vi "PCO_Live.vi"(7 "Message Data":variant, 8 "entrée d'erreur (pas d'erreur)":errorcluster, 9 "Display loop":refnum<queue>, 10 "dup Message Queue":refnum<queue>, 11 "Camera en entrée":refnum<class "Camera.lvclass">) -> (0 "sortie d'erreur":errorcluster, 3 "Camera en sortie":refnum<class "Camera.lvclass">)   [LabVIEW 2026]
uses:
  v0.2/SubVIs/QMH/Message Queue/Message Cluster.ctl
  <instrlib>/PCO_SDK/File Group 0/vi.lib/Excelitas PCO GmbH/pco.labview/camera/Camera.lvclass
  v0.2/SubVIs/Controls/PCO_Config.ctl
  v0.2/SubVIs/Controls/TypeDef_FGV.ctl
  <instrlib>/PCO_SDK/File Group 0/vi.lib/Excelitas PCO GmbH/pco.labview/camera/Controls/binning.ctl
  v0.2/SubVIs/QMH/Message Queue/Enqueue Message (Single).vi
  v0.2/SubVIs/QMH/Message Queue/Message Queue.lvlib
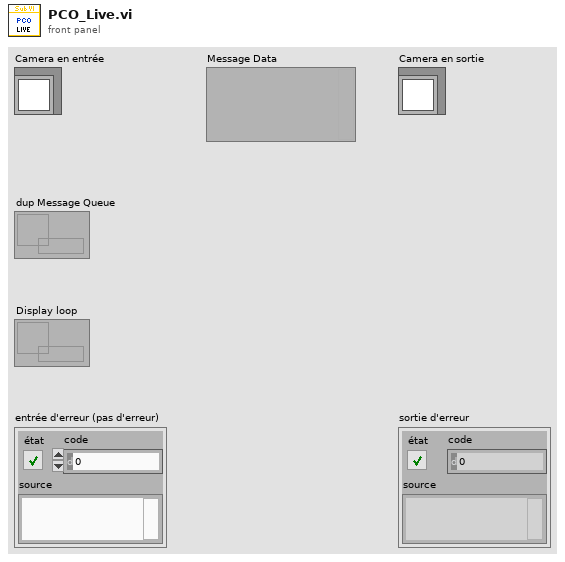
[diagram p1: front panel]
types:
  T1 = typedef "PCO_Config.ctl" = cluster{"Exposure time (s)":dbl, "TriggerMode":u16, "ROI X0":u16, "ROI Y0":u16, "ROI X1":u16, "ROI Y1":u16, "Binning":u8}
  T2 = enum16{"sequence", "sequence non blocking", "ring buffer", "fifo", "sequence_dpcore", "sequence_non_blocking_dpcore", "ring_buffer_dpcore", "fifo_dpcore", "tif", "multitif", "pcoraw", "b16", "dicom", "multidicom", "camram_ring", "camram_segment"}
  T3 = typedef "Camera.lvclass/binning.ctl" = cluster{"vert":u16, "horz":u16, "mode":u16}
  T4 = cluster{"exposure_time_s":dbl, "delay_time_s":dbl, "roi":cluster{"x0":u64, "y0":u64, "x1":u64, "y1":u64}, "timestamp_mode":u16, "pixelrate":u32, "trigger_mode":u16, "acquire_mode":u16, "metadata_mode":u16, "noisefilter_mode":u16, "pixel_format":u32, "binning":T3, "auto_exposure":cluster{"region":u16, "min_exposure_s":dbl, "max_exposure_s":dbl}}
  T5 = typedef "TypeDef_FGV.ctl" = enum16{"Initialize", "Write", "Read"}
  T6 = enum16{"Undefined", "Mono8", "Mono16", "BGRA8", "RGBA8", "BGRA16", "RGBA16", "CompressedMono8"}
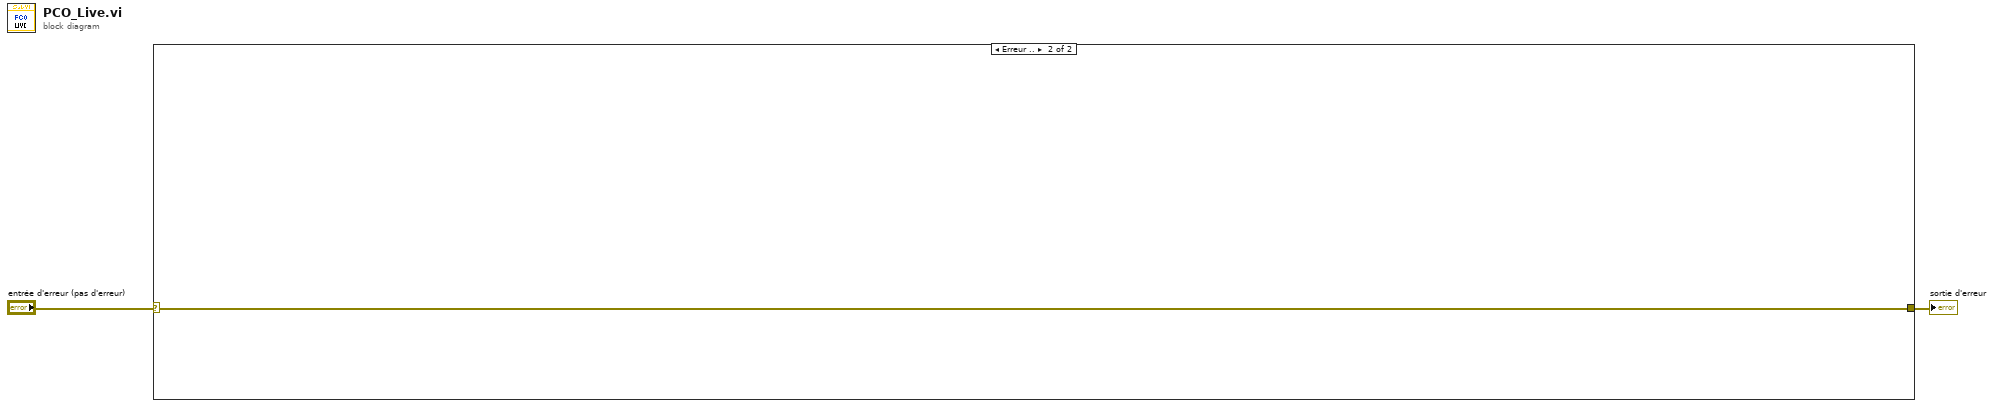
[diagram p0: block diagram]
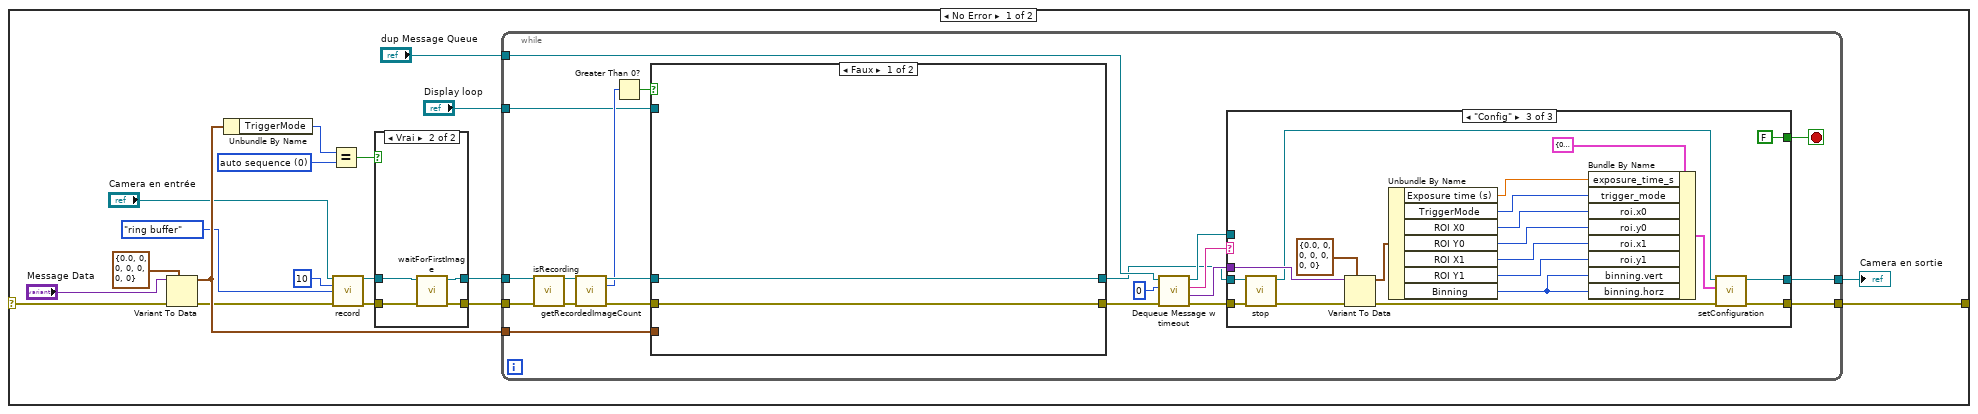
[diagram p2: hidden frame]
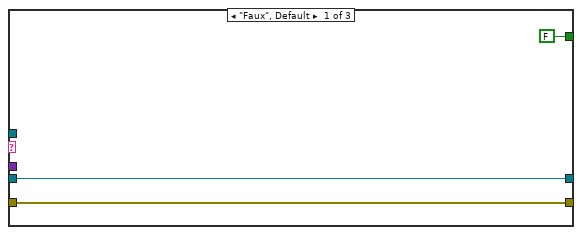
[diagram p3: hidden frame]
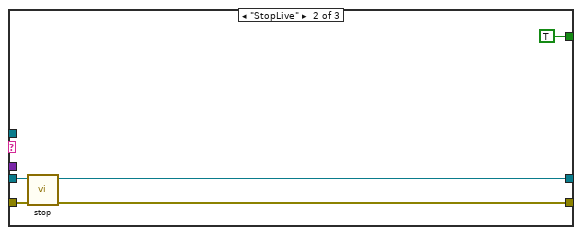
[diagram p4: hidden frame]
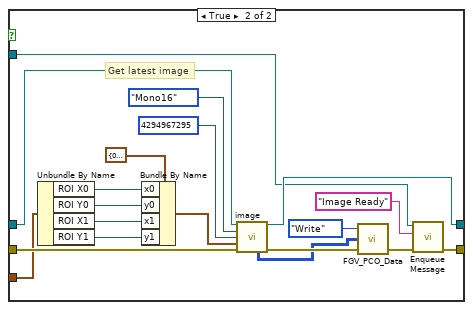
[diagram p5: hidden frame]
diagram:
  n1 = case shown="Erreur .." "entrée d'erreur (pas d'erreur)" {
    selector: "entrée d'erreur (pas d'erreur)" -> [w3 w98]
    tunnel: [w17 w98] -> w2
    frame No Error {
      w9 = u16 0 items=["auto sequence", "software trigger", "external exposure start", "external exposure control"] ("TriggerMode")
      n2 = Variant To Data(error in=w3, type=T1 {"Exposure time (s)"=0.0, "TriggerMode"=0, "ROI X0"=0, "ROI Y0"=0, "ROI X1"=0, "ROI Y1"=0, "Binning"=0} ("PCO_Config"), Variant="Message Data") -> (data=w15:T1, error out=w8:errorcluster)
      n3 = Unbundle By Name(w15) -> ("TriggerMode"=w10:u16)
      n4 = Equal?(x=w10, y=w9) -> (x = y?=w12:bool)
      n5 = call-dynamic "record.vi"("Camera in"="Camera en entrée", "num_images"=u32 10 ("dwImgCount"), "record_mode"=T2."ring buffer", "error in (no error)"=w8) -> ("Camera out"=w20:refnum<class "Camera.lvclass">, "error out"=w19:errorcluster)  [unwired: 10 in]
      n6 = case shown="Vrai" w12 {
        tunnel: w19 -> [w92 w97]
        tunnel: w20 -> [w93 w96]
        tunnel: [w93 w95] -> w14
        tunnel: [w92 w94] -> w13
        frame False {
        }
        frame True {
          n7 = call-dynamic "waitForFirstImage.vi"("error in (no error)"=w97, "Camera in"=w96) -> ("error out"=w94:errorcluster, "Camera out"=w95:refnum<class "Camera.lvclass">)  [unwired: 8 in]
        }
      }
      n8 = while {
        tunnel: w13 -> [w36]
        tunnel: w14 -> [w35]
        tunnel: w15 -> [w34]
        tunnel: "dup Message Queue" -> [w32]
        tunnel: "Display loop" -> [w30]
        tunnel: [w25] -> w17
        tunnel: [w24] -> w18
        stop <- w23 stop-if-true
        n9 = call-dynamic "isRecording.vi"("Camera in"=w35, "error in (no error)"=w36) -> ("Camera out"=w42:refnum<class "Camera.lvclass">, "error out"=w41:errorcluster)  [unwired: 11 in, 1 out]
        n10 = call-dynamic "getRecordedImageCount.vi"("Camera in"=w42, "error in (no error)"=w41) -> ("Camera out"=w39:refnum<class "Camera.lvclass">, "recorded_image_count"=w37:u32, "error out"=w40:errorcluster)  [unwired: 11 in]
        n11 = Greater Than 0?(x=w37) -> (x > 0?=w38:bool)
        n12 = case shown="Faux" w38 {
          tunnel: [w71 w77] -> w33
          tunnel: w40 -> [w71 w88]
          tunnel: w39 -> [w72 w87]
          tunnel: [w72 w86] -> w26
          tunnel: w34 -> [_ w85]
          tunnel: w30 -> [_ w79]
          frame False {
          }
          frame True {
            # "Get latest image"
            n13 = Unbundle By Name(w85) -> ("ROI X0"=w84:u16, "ROI Y0"=w83:u16, "ROI X1"=w82:u16, "ROI Y1"=w81:u16)
            n14 = Bundle By Name(cluster=cluster{"x0":u64, "y0":u64, "x1":u64, "y1":u64} {"x0"=0, "y0"=0, "x1"=0, "y1"=0} ("roi"), "x0"=w84, "y0"=w83, "x1"=w82, "y1"=w81) -> (w89:cluster{"x0":u64, "y0":u64, "x1":u64, "y1":u64})
            n15 = call-dynamic "image.vi"("Camera in"=w87, "data_format"=T6."Mono16", "image_index"=u32 4294967295 ("dwImgIdx"), "roi"=w89, "error in (no error)"=w88) -> ("Camera out"=w86:refnum<class "Camera.lvclass">, "raw_image (U16)"=w73:u16[][], "error out"=w75:errorcluster)  [unwired: 2 in, 6 out]
            n16 = call "FGV_PCO_Data.vi"("error in"=w75, "Data"=w73, "Action"=TypeDef_FGV."Write") -> ("error out"=w74:errorcluster)  [unwired: 1 in, 1 out]
            n17 = call-poly "Enqueue Message.vi"("error in (no error)"=w74, "Message"="Image Ready", "Message Queue"=w79) -> ("error out"=w77:errorcluster)  [unwired: 7 in, 1 out]
          }
        }
        n18 = call "Dequeue Message w timeout.vi"("entrée d'erreur (pas d'erreur)"=w33, "timeout en ms (-1)"=0, "Message Queue"=w32) -> ("sortie d'erreur"=w28:errorcluster, "Message Data"=w27:variant, "Message"=w31:string, "Message Queue"=w29:refnum<queue>)  [unwired: 5 in]
        n19 = case shown="\"Config\"" w31 {
          tunnel: w29 -> [_ _ _]
          tunnel: w28 -> [w44 w49 w69]
          tunnel: w27 -> [_ _ w55]
          tunnel: w26 -> [w45 w50 w70]
          tunnel: [w44 w48 w51] -> w25
          tunnel: [w45 w47 w53] -> w24
          tunnel: [FALSE TRUE FALSE] -> w23
          frame "Faux", Default {
          }
          frame "StopLive" {
            n20 = call-dynamic "stop.vi"("error in (no error)"=w49, "Camera in"=w50) -> ("error out"=w48:errorcluster, "Camera out"=w47:refnum<class "Camera.lvclass">)  [unwired: 8 in]
          }
          frame "Config" {
            n21 = call-dynamic "stop.vi"("error in (no error)"=w69, "Camera in"=w70) -> ("error out"=w54:errorcluster, "Camera out"=w52:refnum<class "Camera.lvclass">)  [unwired: 8 in]
            n22 = Variant To Data(error in=w54, type=T1 {"Exposure time (s)"=0.0, "TriggerMode"=0, "ROI X0"=0, "ROI Y0"=0, "ROI X1"=0, "ROI Y1"=0, "Binning"=0} ("PCO_Config"), Variant=w55) -> (data=w67:T1, error out=w66:errorcluster)
            n23 = Unbundle By Name(w67) -> ("Exposure time (s)"=w64:dbl, "TriggerMode"=w63:u16, "ROI X0"=w58:u16, "ROI Y0"=w59:u16, "ROI X1"=w60:u16, "ROI Y1"=w61:u16, "Binning"=w62:u8)
            n24 = Bundle By Name(cluster=T4 {"exposure_time_s"=0.1, "delay_time_s"=nan, "roi"={"x0"=18446744073709551615, "y0"=18446744073709551615, "x1"=18446744073709551615, "y1"=18446744073709551615}, "timestamp_mode"=65535, "pixelrate"=4294967295, "trigger_mode"=65535, "acquire_mode"=65535, "metadata_mode"=65535, "noisefilter_mode"=65535, "pixel_format"=4294967295, "binning"={"vert"=65535, "horz"=65535, "mode"=0}, "auto_exposure"={"region"=0, "min_exposure_s"=0.001, "max_exposure_s"=0.1}} ("configuration"), "exposure_time_s"=w64, "trigger_mode"=w63, "roi.x0"=w58, "roi.y0"=w59, "roi.x1"=w60, "roi.y1"=w61, "binning.vert"=w62, "binning.horz"=w62) -> (w65:T4)
            n25 = call-dynamic "setConfiguration.vi"("error in (no error)"=w66, "configuration"=w65, "Camera in"=w52) -> ("error out"=w51:errorcluster, "Camera out"=w53:refnum<class "Camera.lvclass">)  [unwired: 7 in]
          }
        }
      }
      "Camera en sortie" <- w18
    }
    frame Error {
    }
  }
  "sortie d'erreur" <- w2
